vi "Latihan 14 (SubVI_2).vi"() -> ()   [LabVIEW 2021]
panel:
  out "R":dbl(slide) scale=0.0..80.0
  out "K":dbl(slide) scale=273.15..373.15
  in  "Convert":bool
  out "C":dbl(slide) scale=0.0..100.0
  in  "F":dbl(slide) scale=32.0..212.0
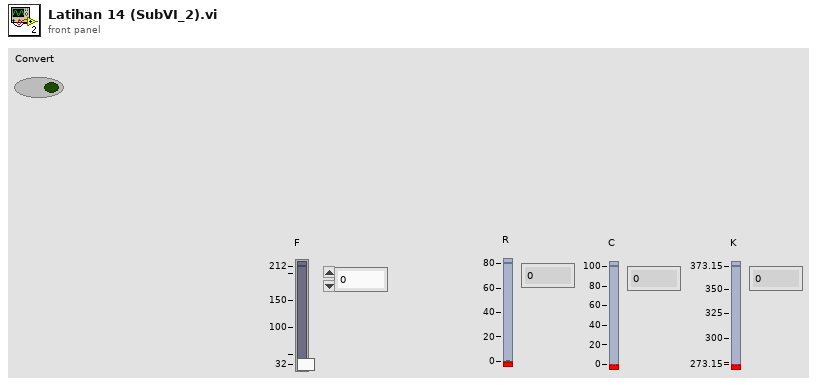
[diagram p1: front panel]
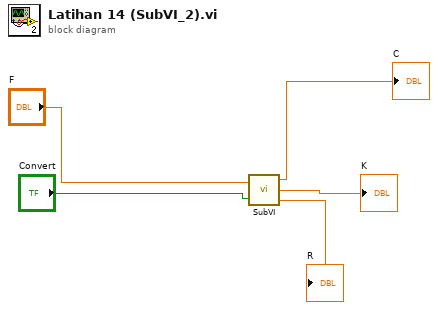
[diagram p0: block diagram]
diagram:
  n1 = call "SubVI.vi"("F"="F", "Convert"="Convert") -> ("Celcius"=→"C":dbl, "Kelvin"=→"K":dbl, "Reamur"=→"R":dbl)
